vi "Main Page.vi"(8 "error in (no error)":errorcluster, 11 "Node Ptr":T1 format="%.0x") -> (0 "error out":errorcluster)   [LabVIEW 2017, in "PXImc System Explorer.lvlib"]
uses:
  PXImc System Explorer.lvlib
  <vilib>/NI Veristand/Custom Device API/Custom Device Item Ref.ctl
  Shared/Constants.vi
  <vilib>/NI Veristand/Custom Device API/Get Item Property (String).vi
  <vilib>/NI Veristand/Custom Device API/Get Item Property (U16).vi
  <vilib>/NI Veristand/Custom Device API/Set Item Property (String).vi
  <vilib>/NI Veristand/Custom Device API/Set Item Property (U16).vi
  <vilib>/NI VeriStand/Custom Device API/Custom Device API.lvlib
  Shared/PXImc Shared.lvlib
  Utility/Import Export - Configuration Dialog.vi
panel:
  out "Version":string
  in  "Module Name":string
  in  "Remote write ID":u16
  in  "My write ID":u16
  in  "Header":cluster{"Section Name":string}={"Section Name"="PXImc Custom Device Settings"}
  in  "Description":string
  in  "Name":string
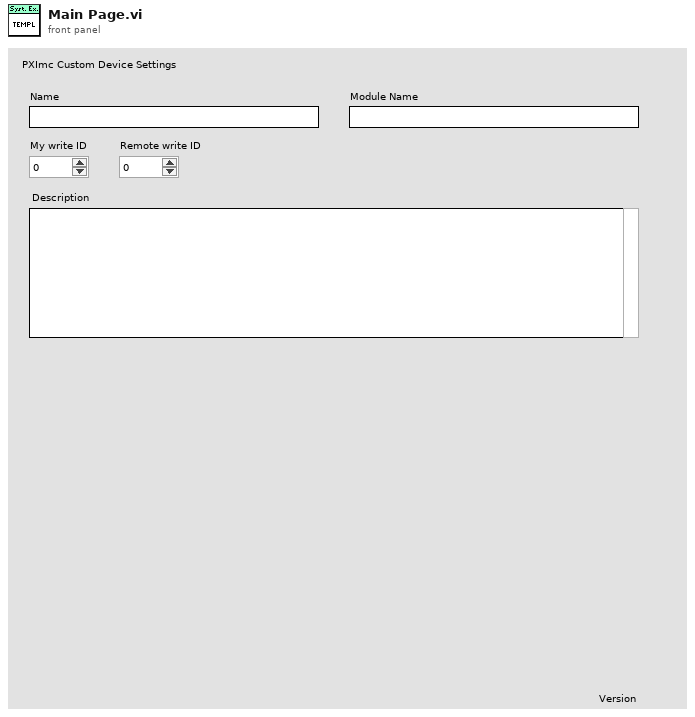
[diagram p1: front panel]
types:
  T1 = typedef "Custom Device API.lvlib/Custom Device Item Ref.ctl" = u64
  T2 = typedef "Custom Device API.lvlib/Custom Device Item Info.ctl" = cluster{"Name":string, "Is Channel":bool, "GUID":string, "Is Waveform":bool}
  T3 = typedef "Custom Device API.lvlib/Custom Device Commands.ctl" = enum16{"Default", "Item renamed", "Shutdown", "Dynamic button pressed"}
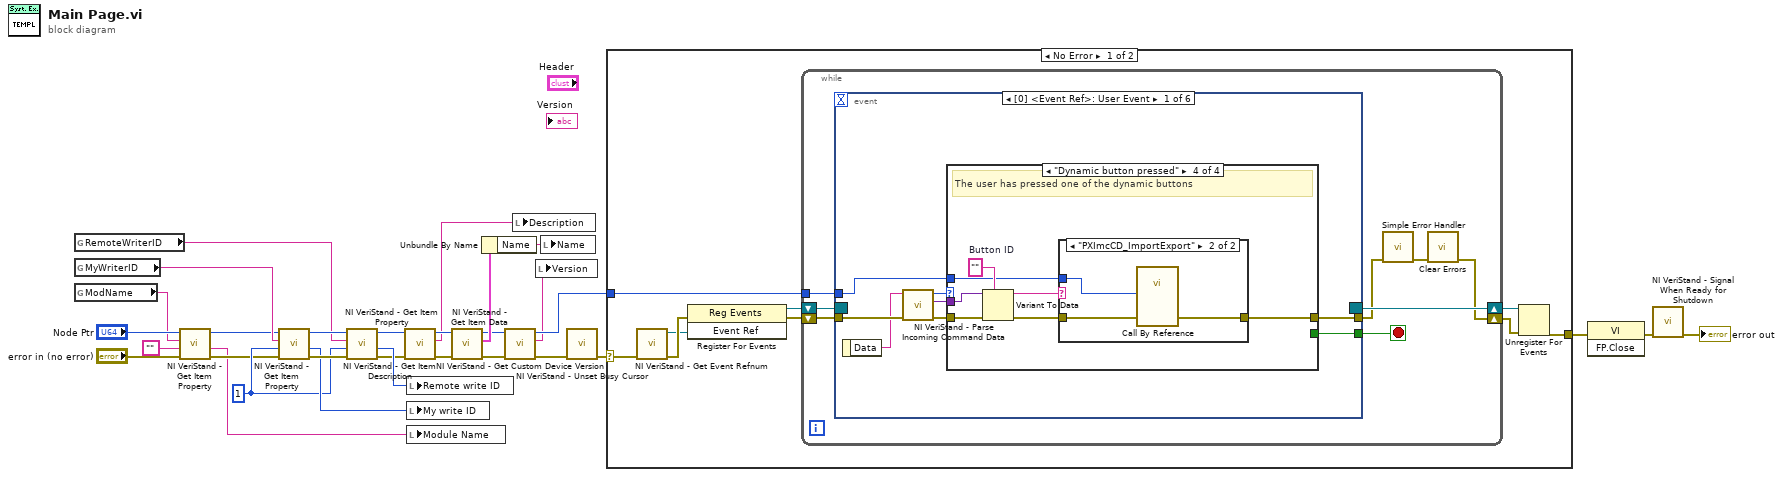
[diagram p0: block diagram]
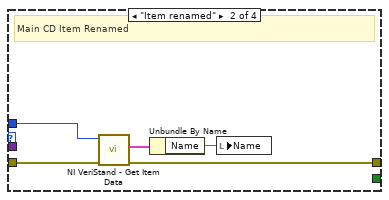
[diagram p3: hidden frame]
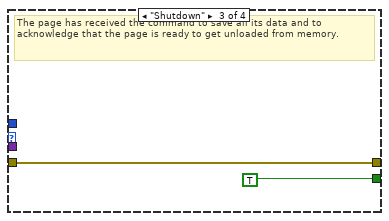
[diagram p4: hidden frame]
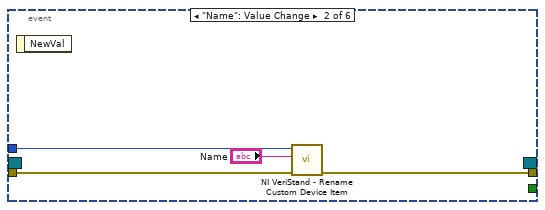
[diagram p6: hidden frame]
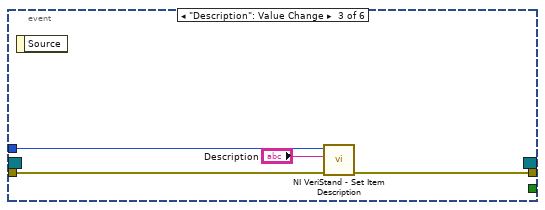
[diagram p7: hidden frame]
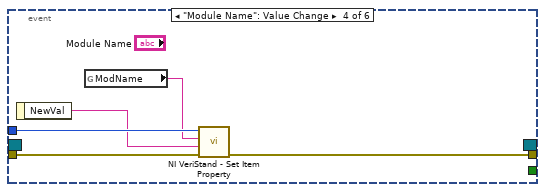
[diagram p8: hidden frame]
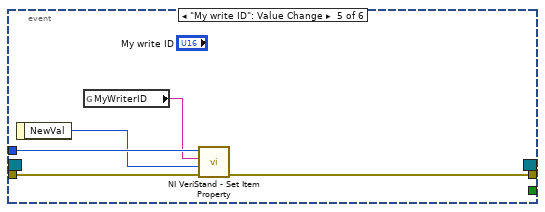
[diagram p9: hidden frame]
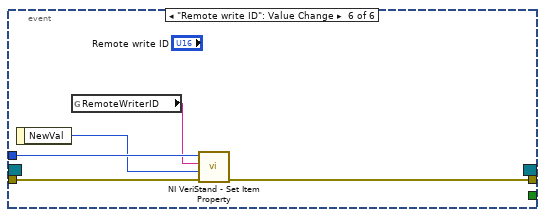
[diagram p10: hidden frame]
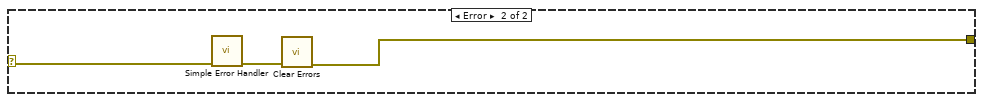
[diagram p11: hidden frame]
diagram:
  w15 = u16 1 ("Default Value")
  n1 = global read "Constants.vi" "RemoteWriterID"() -> (w17:string)
  n2 = global read "Constants.vi" "MyWriterID"() -> (w19:string)
  n3 = global read "Constants.vi" "ModName"() -> (w8:string)
  n4 = call-poly <vilib>:"NI VeriStand - Get Item Property.vi"("error in (no error)"="error in (no error)", "Default Value"="", "Property Name"=w8, "Item Ref in"="Node Ptr") -> ("error out"=w11:errorcluster, "Value"=w6:string, "Item Ref out"=w9:T1)  [unwired: 4 in, 1 out]
  n5 = call-poly <vilib>:"NI VeriStand - Get Item Property.vi"("error in (no error)"=w11, "Default Value"=w15, "Property Name"=w19, "Item Ref in"=w9) -> ("error out"=w20:errorcluster, "Value"=w16:u16, "Item Ref out"=w18:T1)  [unwired: 4 in, 1 out]
  n6 = call-poly <vilib>:"NI VeriStand - Get Item Property.vi"("error in (no error)"=w20, "Default Value"=w15, "Property Name"=w17, "Item Ref in"=w18) -> ("error out"=w12:errorcluster, "Value"=w14:u16, "Item Ref out"=w13:T1)  [unwired: 4 in, 1 out]
  n7 = call <vilib>:"NI VeriStand - Get Item Description.vi"("error in (no error)"=w12, "Item Ref in"=w13) -> ("error out"=w24:errorcluster, "Description"=w25:string, "Item Ref out"=w26:T1)  [unwired: 7 out]
  n8 = local write "Remote write ID"(w14) -> ()
  n9 = local write "My write ID"(w16) -> ()
  n10 = local write "Module Name"(w6) -> ()
  n11 = call <vilib>:"NI VeriStand - Get Item Data.vi"("error in (no error)"=w24, "Item Ref in"=w26) -> ("error out"=w5:errorcluster, "Item Info"=w23:T2, "Item Ref out"=w4:T1)  [unwired: 7 out]
  n12 = Unbundle By Name(w23) -> ("Name"=w22:string)
  n13 = call <vilib>:"NI VeriStand - Get Custom Device Version.vi"("error in (no error)"=w5, "Device Ref in"=w4) -> ("error out"=w2:errorcluster, "Value"=w1:string, "Device Ref out"=w3:T1)  [unwired: 7 in]
  n14 = local write "Description"(w25) -> ()
  n15 = local write "Version"(w1) -> ()
  n16 = local write "Name"(w22) -> ()
  n17 = call <vilib>:"NI VeriStand - Unset Busy Cursor.vi"("error in (no error)"=w2) -> ("error out"=w27:errorcluster)  [unwired: 10 out]
  n18 = case shown="No Error" w27 {
    selector: w27 -> [w32 w100]
    tunnel: [w36 w98] -> w30
    tunnel: w3 -> [w31 _]
    frame No Error {
      n19 = call <vilib>:"NI VeriStand - Get Event Refnum.vi"("error in (no error)"=w32) -> ("error out"=w39:errorcluster, "Event Ref"=w35:refnum<user-event>)  [unwired: 9 out]
      n20 = register-events(error in=w39, w35) -> (reference out=w33:refnum<event-registration>, error out=w34:errorcluster)  [unwired: 1 in]
      n21 = while {
        shift-right: [w42] -> w37
        shift-left: w34 -> [w46]
        shift-right: [w47] -> w38
        shift-left: w33 -> [w45]
        tunnel: w31 -> [w40]
        stop <- w44 stop-if-true
        n22 = event shown="[0] <Event Ref>: User Event" {
          selector: w45 -> [_ _ _ _ _ _]
          dyn-events: [_ _ _ _ _ _] -> w47
          timeout: _ -> [_ _ _ _ _ _]
          tunnel: w46 -> [w55 w78 w82 w87 w92 w97]
          tunnel: [w52 _ _ _ _ _] -> w44
          tunnel: [w51 w77 w81 w85 w90 w95] -> w41
          tunnel: w40 -> [w49 w75 w79 w86 w91 w96]
          event User Event {
            n23 = event-data() -> ("Data"=w48:string)  [unwired: 1 out]
            n24 = call <vilib>:"NI VeriStand - Parse Incoming Command Data.vi"("error in (no error)"=w55, "Incoming data"=w48) -> ("error out"=w54:errorcluster, "Outgoing data"=w50:variant, "Action"=w53:T3)  [unwired: 7 out]
            n25 = case shown="\"Dynamic button pressed\"" w53 {
              tunnel: w54 -> [w56 w61 w62 w70]
              tunnel: [_ _ TRUE _] -> w52
              tunnel: [w56 w59 w62 w66] -> w51
              tunnel: w50 -> [_ _ _ w69]
              tunnel: w49 -> [_ w57 _ w64]
              frame "Default", Default {
              }
              frame "Item renamed" {
                # "Main CD Item Renamed"
                n26 = call <vilib>:"NI VeriStand - Get Item Data.vi"("error in (no error)"=w61, "Item Ref in"=w57) -> ("error out"=w59:errorcluster, "Item Info"=w60:T2)  [unwired: 8 out]
                n27 = Unbundle By Name(w60) -> ("Name"=w58:string)
                n28 = local write "Name"(w58) -> ()
              }
              frame "Shutdown" {
                # "The page has received the command to save all its data and to acknowledge that the page is ready to get unloaded from memory."
              }
              frame "Dynamic button pressed" {
                w68 = ""  # Button ID
                # "The user has pressed one of the dynamic buttons"
                n29 = Variant To Data(error in=w70, type=w68, Variant=w69) -> (data=w65:string, error out=w67:errorcluster)
                n30 = case shown="\"PXImcCD_ImportExport\"" w65 {
                  tunnel: w67 -> [w71 w74]
                  tunnel: [w71 w73] -> w66
                  tunnel: w64 -> [_ w72]
                  frame Default {
                  }
                  frame "PXImcCD_ImportExport" {
                    n31 = call-by-ref "?"("error in"=w74, "Item Ref in"=w72) -> ("error out"=w73:errorcluster)  [unwired: 10 in, 3 out]
                  }
                }
              }
            }
          }
          event "Name": Value Change {
            n32 = event-data() -> ()  [unwired: 2 out]
            n33 = call <vilib>:"NI VeriStand - Rename Custom Device Item.vi"("error in (no error)"=w78, "New Name"="Name", "Item Ref in"=w75) -> ("error out"=w77:errorcluster)  [unwired: 1 in, 7 out]
          }
          event "Description": Value Change {
            n34 = event-data() -> ()  [unwired: 2 out]
            n35 = call <vilib>:"NI VeriStand - Set Item Description.vi"("error in (no error)"=w82, "Description"="Description", "Item Ref in"=w79) -> ("error out"=w81:errorcluster)  [unwired: 8 out]
          }
          event "Module Name": Value Change {
            n36 = event-data() -> ("NewVal"=w84:string)  [unwired: 1 out]
            n37 = global read "Constants.vi" "ModName"() -> (w83:string)
            n38 = call-poly <vilib>:"NI VeriStand - Set Item Property.vi"("error in (no error)"=w87, "Value"=w84, "Property Name"=w83, "Item Ref in"=w86) -> ("error out"=w85:errorcluster)  [unwired: 5 in, 2 out]
          }
          event "My write ID": Value Change {
            n39 = event-data() -> ("NewVal"=w89:u16)  [unwired: 1 out]
            n40 = global read "Constants.vi" "MyWriterID"() -> (w88:string)
            n41 = call-poly <vilib>:"NI VeriStand - Set Item Property.vi"("error in (no error)"=w92, "Value"=w89, "Property Name"=w88, "Item Ref in"=w91) -> ("error out"=w90:errorcluster)  [unwired: 5 in, 2 out]
          }
          event "Remote write ID": Value Change {
            n42 = event-data() -> ("NewVal"=w94:u16)  [unwired: 1 out]
            n43 = global read "Constants.vi" "RemoteWriterID"() -> (w93:string)
            n44 = call-poly <vilib>:"NI VeriStand - Set Item Property.vi"("error in (no error)"=w97, "Value"=w94, "Property Name"=w93, "Item Ref in"=w96) -> ("error out"=w95:errorcluster)  [unwired: 5 in, 2 out]
          }
        }
        n45 = call <vilib>:"Simple Error Handler.vi"("error in (no error)"=w41) -> ("error out"=w43:errorcluster)  [unwired: 1 in, 7 out]
        n46 = call <vilib>:"Clear Errors.vi"("error in (no error)"=w43) -> ("error out"=w42:errorcluster)  [unwired: 1 in, 5 out]
      }
      n47 = Unregister For Events(event registration refnum=w38, error in=w37) -> (error out=w36:errorcluster)
    }
    frame Error {
      n48 = call <vilib>:"Simple Error Handler.vi"("error in (no error)"=w100) -> ("error out"=w99:errorcluster)  [unwired: 1 in, 7 out]
      n49 = call <vilib>:"Clear Errors.vi"("error in (no error)"=w99) -> ("error out"=w98:errorcluster)  [unwired: 1 in, 5 out]
    }
  }
  n50 = invoke class="VI" method="FP.Close"(error in=w30) -> (error out=w29:errorcluster)  [unwired: 2 in, 2 out]
  n51 = call <vilib>:"NI VeriStand - Signal When Ready for Shutdown.vi"("error in (no error)"=w29) -> ("error out"=→"error out":errorcluster)  [unwired: 10 out]
